vi "File System Query.vi"(8 "error in (no error)":errorcluster, 11 "VISA resource name":refnum<visa-resource-name>) -> (0 "error out":errorcluster, 1 "Folder Names":string[](array[string]), 2 "Filenames":string[](array[string]), 3 "VISA resource name out":refnum<visa-resource-name>, 4 "Free Space (Byte)":dbl, 5 "Current Working Directory":string)   [LabVIEW 2016, in "Tektronix DPO MSO 2000 4000 Series.lvlib"]
doc: "Queries the oscilloscope for file system commands."
uses:
  Tektronix DPO MSO 2000 4000 Series.lvlib
  <vilib>/regexp/Match Regular Expression.xnode
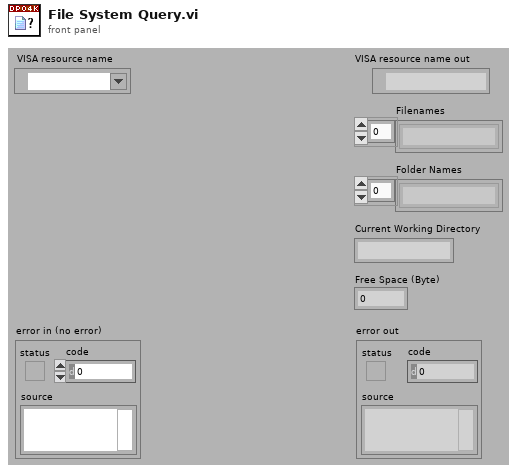
[diagram p1: front panel]
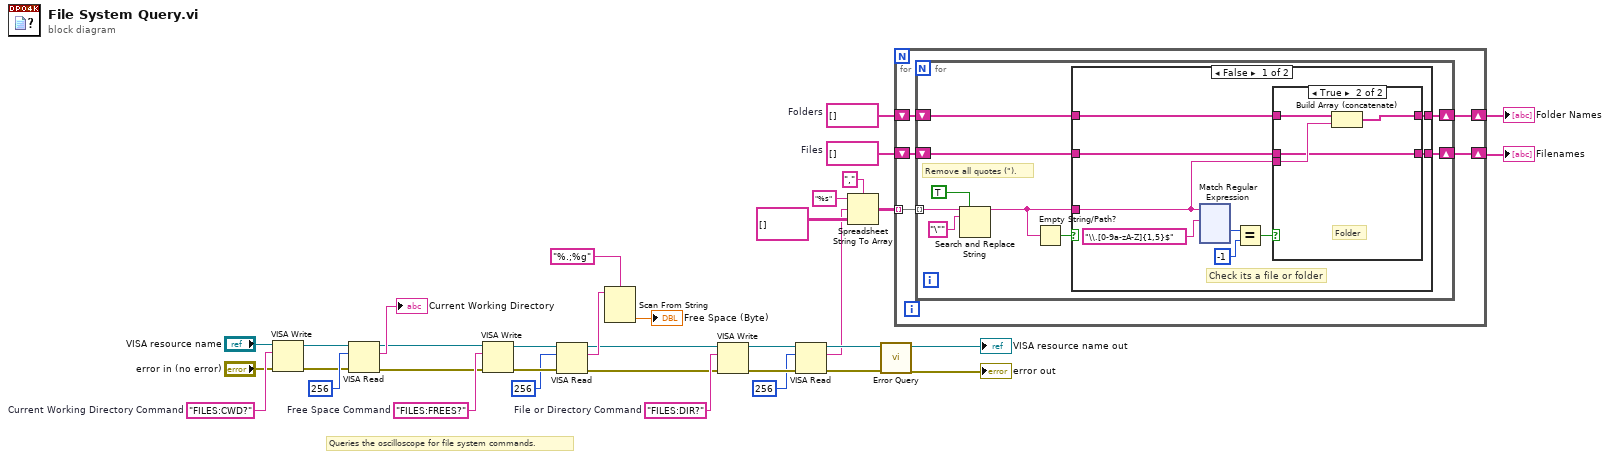
[diagram p0: block diagram]
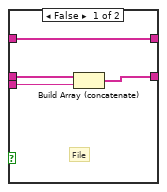
[diagram p2: hidden frame]
diagram:
  w15 = string[] []  # Files
  w14 = string[] []  # Folders
  w24 = "FILES:FREES?"  # Free Space Command
  w26 = "FILES:CWD?"  # Current Working Directory Command
  w35 = "FILES:DIR?"  # File or Directory Command
  # "Queries the oscilloscope for file system commands."
  n1 = VISA Write(VISA resource name="VISA resource name", write buffer=w26, error in (no error)="error in (no error)") -> (VISA resource name out=w27:refnum<visa-resource-name>, error out=w28:errorcluster)  [unwired: 1 out]
  n2 = VISA Read(VISA resource name=w27, byte count=u32 256, error in (no error)=w28) -> (VISA resource name out=w19:refnum<visa-resource-name>, read buffer=→"Current Working Directory":string, error out=w20:errorcluster)  [unwired: 1 out]
  n3 = VISA Write(VISA resource name=w19, write buffer=w24, error in (no error)=w20) -> (VISA resource name out=w23:refnum<visa-resource-name>, error out=w22:errorcluster)  [unwired: 1 out]
  n4 = VISA Read(VISA resource name=w23, byte count=u32 256, error in (no error)=w22) -> (VISA resource name out=w7:refnum<visa-resource-name>, read buffer=w18:string, error out=w5:errorcluster)  [unwired: 1 out]
  n5 = Scan From String(format string="%.;%g", input string=w18) -> (output 1=→"Free Space (Byte)":dbl)  [unwired: 3 in, 3 out]
  n6 = VISA Write(VISA resource name=w7, write buffer=w35, error in (no error)=w5) -> (VISA resource name out=w32:refnum<visa-resource-name>, error out=w31:errorcluster)  [unwired: 1 out]
  n7 = VISA Read(VISA resource name=w32, byte count=u32 256, error in (no error)=w31) -> (VISA resource name out=w6:refnum<visa-resource-name>, read buffer=w3:string, error out=w4:errorcluster)  [unwired: 1 out]
  n8 = Spreadsheet String To Array(delimiter (Tab)=",", format string="%s", spreadsheet string=w3, array type (2D Dbl)=string[][] [] ("array")) -> (array=w13:string[][])
  n9 = call "Error Query.vi"("error in (no error)"=w4, "VISA resource name"=w6) -> ("error out"=→"error out":errorcluster, "VISA resource name out"=→"VISA resource name out":refnum<visa-resource-name>)  [unwired: 6 in, 2 out]
  n10 = for {
    tunnel: w13 -> [w40] mode=indexing
    shift-right: [w38] -> w2
    shift-left: w14 -> [w39]
    shift-right: [w36] -> w1
    shift-left: w15 -> [w37]
    n11 = for {
      tunnel: w40 -> [w47] mode=indexing
      shift-right: [w45] -> w38
      shift-left: w39 -> [w46]
      shift-right: [w43] -> w36
      shift-left: w37 -> [w44]
      # "Remove all quotes (\")."
      n12 = Search and Replace String(replace all?=TRUE ("replace all? (F)"), input string=w47, search string="\"") -> (result string=w42:string)  [unwired: 5 in, 3 out]
      n13 = Empty String/Path?(string/path=w42) -> (empty?=w41:bool)
      n14 = case shown="False" w41 {
        tunnel: w46 -> [w54 w182]
        tunnel: [w53 w182] -> w45
        tunnel: w44 -> [w52 w181]
        tunnel: [w51 w181] -> w43
        tunnel: w42 -> [w50 _]
        frame False {
          # "Check its a file or folder"
          n15 = xnode "Match Regular Expression"("input string"=w50, "regular expression"="\\.[0-9a-zA-Z]{1,5}$") -> ("offset past match"=w57:i32)  [unwired: 4 in, 4 out]
          n16 = Equal?(x=w57, y=-1) -> (x = y?=w55:bool)
          n17 = case shown="True" w55 {
            tunnel: w54 -> [w62 w66]
            tunnel: w50 -> [w59 w65]
            tunnel: [w62 w64] -> w53
            tunnel: w52 -> [w61 w63]
            tunnel: [w60 w63] -> w51
            frame False {
              # "File"
              n18 = Build Array (concatenate)(w61, w59) -> (w60:string[])
            }
            frame True {
              # "Folder"
              n19 = Build Array (concatenate)(w66, w65) -> (w64:string[])
            }
          }
        }
        frame True {
        }
      }
    }
  }
  "Filenames" <- w1
  "Folder Names" <- w2
